vi "sub_VI_Fourier_series_EMF.vi"(10 "del t":dbl, 11 "x,i":dbl[](array[numeric])=[1.388528617422219e-06, 1.0215603399606325e-05, 2.122465172345392e-05, 2.9975433724460983e-05, 3.867281077864411e-05, 4.72938950516502e-05, 5.581579870912612e-05, 6.427666814166041e-05, 7.25773227337229e-05, 8.279292613332924e-05, 9.083418526938979e-05, 9.869234173062542e-05, 0.00010644368829821318, 0.00011401193219097605, 0.00012141233196514943, 0.00013043013870027613, 0.0001374490745685643, 0.000144246761371439, 0.00015087660405572418, 0.00015725468056212516, 0.0001634343958374658, 0.00017082716633352147, 0.0001764575735843874, 0.00018186673176983988, 0.0001870088652211727, 0.0001918916032165036, 0.0001964996871995971, 0.00020187832827257878, 0.00020583792361566743, 0.00020953049422463643, 0.00021290263515266178, 0.00021600012206844982, 0.00021877717930329427, 0.00022182889055037604, 0.00022393457131086248, 0.00022571219311228765, 0.0002271693852327692, 0.00022831377695042488, 0.00022915299754337239, 0.0002297175641240825, 0.0002298320032958481, 0.00022961075423043466, 0.00022907670476219534, 0.0002281917085005416, 0.00022703968750476824, 0.00022510185086287127, 0.00022320216061156285, 0.0002209972992355463, 0.0002184796374567038, 0.0002156262874406823, 0.00021249065413430574, 0.0002081495948853319, 0.00020434258510459733, 0.0002002532920335077, 0.00019590460350641617, 0.00019124311457649872, 0.00018631460091246161, 0.00017981445595617737, 0.00017432137571143013, 0.00016859178784503406, 0.00016261043380075372, 0.00015642308924729536, 0.00014998397851595277, 0.00014168332392389027, 0.00013484749073042703, 0.0001278056670277858, 0.00012060362848467275, 0.0001132413751010879, 0.00010574179471138436, 9.618230922990063e-05, 8.836229915925353e-05, 8.042784991684085e-05, 7.23713322245449e-05, 6.420800463860107e-05, 5.5907350046538575e-05, 4.540183407845948e-05, 3.689518897721896e-05, 2.8358026763507628e-05, 1.976745960297236e-05, 1.1115858217495457e-05, 2.4795153882539626e-06, -8.315913148297907e-06, -1.6944626699421696e-05, -2.5519935303721554e-05, -3.404183896119748e-05, -4.248744983749636e-05, -5.08643972107359e-05, -6.122495689457861e-05, -6.940354303675784e-05, -7.74524314509361e-05, -8.537925141523107e-05, -9.318400292964277e-05, -0.00010089720310664201, -0.00011030410302577168, -0.00011762821001876798, -0.00012482261928376334, -0.00013182629659581606, -0.0001386392419549262, -0.00014523093824862286, -0.00015323405099409488, -0.00015937561987884702, -0.00016531882753253882, -0.0001710102690083464, -0.00017646520286250509, -0.00018166837053877957, -0.0001878251979797671, -0.00019247142835344914, -0.0001968277461586584, -0.000200917039229748, -0.00020473167828860027, -0.00020824114622274435, -0.00021223125867830377, -0.00021507697941620756, -0.0002176327875856386, -0.00021989105390847913, -0.00022182126127225833, -0.0002234691853456825, -0.00022507896302851815, -0.0002259944764026427, -0.00022660481865205908, -0.00022687947266429644, -0.0002268260677174725, -0.0002264827502021758, -0.00022559775394052206, -0.00022453728428216115, -0.0002231106092741504, -0.00022140928025390233, -0.00021936463371835752, -0.0002169995575018691, -0.0002135816409051375, -0.00021052992965805566, -0.0002071577887300303, -0.00020349573523353214, -0.0001995285106123258, -0.0001952713734226467, -0.00018956467339060373, -0.00018468193539527284, -0.0001795321726658223, -0.00017415353159284063, -0.00016846209011703306, -0.0001625570288539298, -0.00015486671651128366, -0.00014841234722370565, -0.00014176724598318502, -0.00013492378351160408, -0.0001278590719746097, -0.00012059599920655504, -0.00011128065062483784, -0.00010359796756030941, -9.580847460213311e-05, -8.784350824724962e-05, -7.973358560812974e-05, -7.149396524100888e-05, -6.105711277598912e-05, -5.258098478721941e-05, -4.401330546103726e-05, -3.539222118803118e-05, -2.670247341196575e-05, -1.7974579245311805e-05, -7.0036773120527314e-06]) -> (3 "computed amplitude":dbl)   [LabVIEW 2018]
panel:
  out "a":dbl
  out "b":dbl
  out "Time period":dbl
  out "N":i32
  out "number of cycles":dbl
  out "t,i":dbl[](array[numeric])
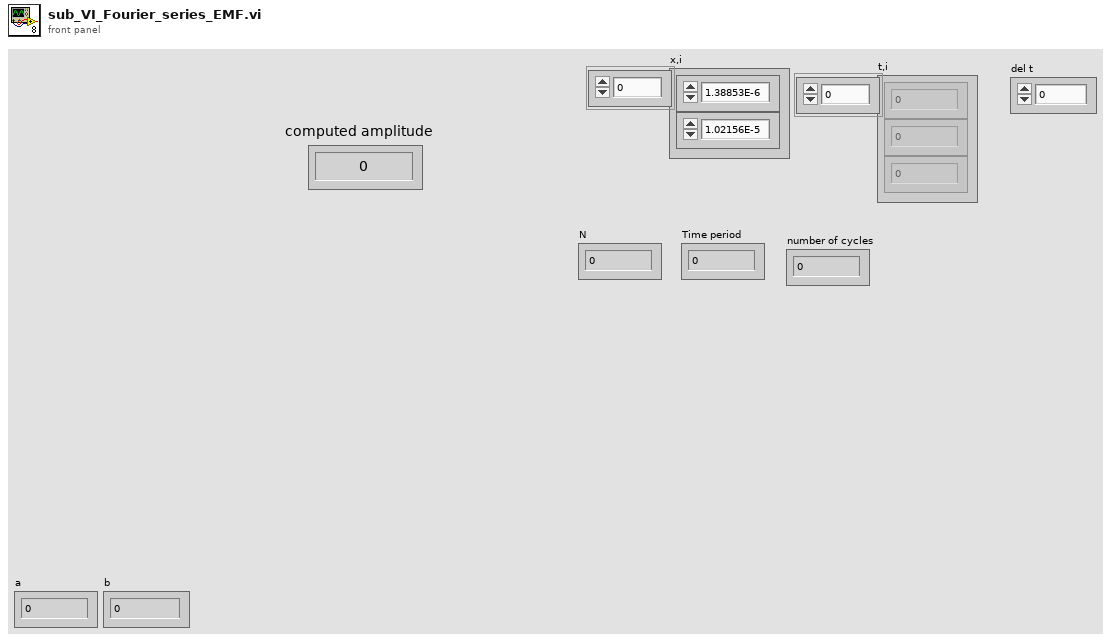
[diagram p1: front panel]
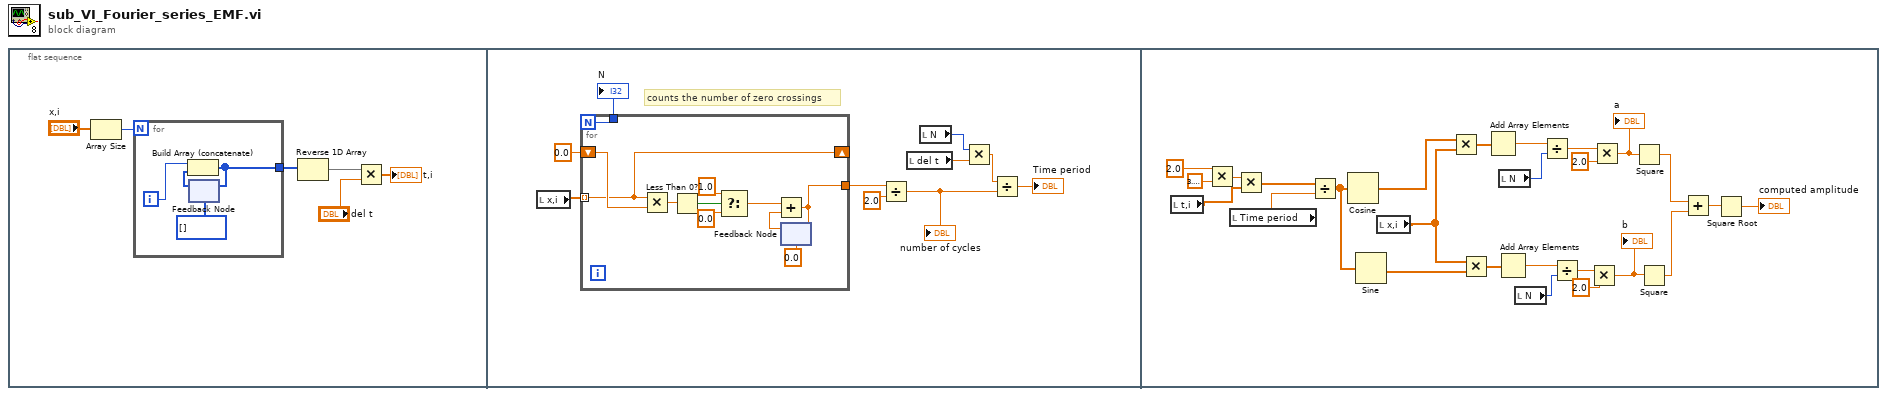
[diagram p0: block diagram]
diagram:
  n1 = flat-sequence {
    frame #0 {
      n2 = Array Size(array="x,i") -> (size(s)=w3:i32)
      n3 = for {
        N: w3 -> [_]
        tunnel: [w7] -> w6
        i -> [w10]
        n4 = feedback #1(i32[] []) -> (w9:i32[])
        n5 = Build Array (concatenate)(w10, w9) -> (w7:i32[])
        n6 = feedback-in #1(w7) -> ()
      }
      n7 = Reverse 1D Array(array=w6) -> (reversed array=w5:i32[])
      n8 = Multiply(x=w5, y="del t") -> (x*y=→"t,i":dbl[])
    }
    frame #1 {
      # "counts the number of zero crossings"
      n9 = local read "x,i"() -> (w13:dbl[])
      n10 = for {
        N -> [w22]
        tunnel: w13 -> [w21] mode=indexing
        tunnel: [w24] -> w18
        shift-right: [w21] -> _
        shift-left: 0.0 ("Numeric Control") -> [w23]
        tunnel: [w22] -> w19
        n11 = Multiply(x=w21, y=w23) -> (x*y=w31:dbl)
        n12 = Less Than 0?(x=w31) -> (x < 0?=w30:bool)
        n13 = Select(t=1.0, s=w30, f=0.0) -> (s? t:f=w27:dbl)
        n14 = feedback #2(0.0) -> (w26:dbl)
        n15 = Add(x=w27, y=w26) -> (x+y=w24:dbl)
        n16 = feedback-in #2(w24) -> ()
      }
      "N" <- w19
      n17 = Divide(x=w18, y=2.0) -> (x/y=w14:dbl)
      "number of cycles" <- w14
      n18 = local read "del t"() -> (w16:dbl)
      n19 = local read "N"() -> (w17:i32)
      n20 = Multiply(x=w17, y=w16) -> (x*y=w15:dbl)
      n21 = Divide(x=w15, y=w14) -> (x/y=→"Time period":dbl)
    }
    frame #2 {
      n22 = local read "t,i"() -> (w51:dbl[])
      n23 = Multiply(x=2.0, y=3.141592653589793) -> (x*y=w36:dbl)
      n24 = local read "Time period"() -> (w52:dbl)
      n25 = Multiply(x=w36, y=w51) -> (x*y=w37:dbl[])
      n26 = Divide(x=w37, y=w52) -> (x/y=w41:dbl[])
      n27 = Cosine(x=w41) -> (cos(x)=w56:dbl[])
      n28 = Sine(x=w41) -> (sin(x)=w55:dbl[])
      n29 = local read "x,i"() -> (w57:dbl[])
      n30 = Multiply(x=w56, y=w57) -> (x*y=w38:dbl[])
      n31 = Multiply(x=w57, y=w55) -> (x*y=w42:dbl[])
      n32 = Add Array Elements(numeric array=w38) -> (sum=w39:dbl)
      n33 = Add Array Elements(numeric array=w42) -> (sum=w43:dbl)
      n34 = local read "N"() -> (w53:i32)
      n35 = local read "N"() -> (w54:i32)
      n36 = Divide(x=w39, y=w53) -> (x/y=w40:dbl)
      n37 = Divide(x=w43, y=w54) -> (x/y=w44:dbl)
      n38 = Multiply(x=w44, y=2.0) -> (x*y=w46:dbl)
      "b" <- w46
      n39 = Multiply(x=w40, y=2.0) -> (x*y=w45:dbl)
      "a" <- w45
      n40 = Square(x=w45) -> (x^2=w47:dbl)
      n41 = Square(x=w46) -> (x^2=w48:dbl)
      n42 = Add(x=w47, y=w48) -> (x+y=w49:dbl)
      n43 = Square Root(x=w49) -> (sqrt(x)=→"computed amplitude":dbl)
    }
  }
